vi "Init.vi"(7 "I2C #":T2=-1, 8 "error in (no error)":errorcluster, 9 "Address":T1=48 format="%02x", 10 "Session In":refnum<class "Session.lvclass">) -> (0 "error out":errorcluster, 3 "Grove I2C Matrix LED Driver Out":refnum<class "Grove I2C Matrix LED Driver.lvclass">)   [LabVIEW 2020, in "CTI-Peripheral.lvlib" / "Grove I2C Matrix LED Driver.lvclass"]
uses:
  Grove I2C Matrix LED Driver.lvclass
  CTI/I2C Connection/I2C Connection.lvclass/I2C Connection.ctl
  Grove I2C Matrix LED Driver.lvclass/Grove I2C Matrix LED Driver.ctl
  CTI/I2C Connection/I2C Connection.lvclass
  CTI/Session/Session.lvclass
  CTI/I2C Number.ctl
  CTI/CTI.lvlib
  CTI/I2C Address.ctl
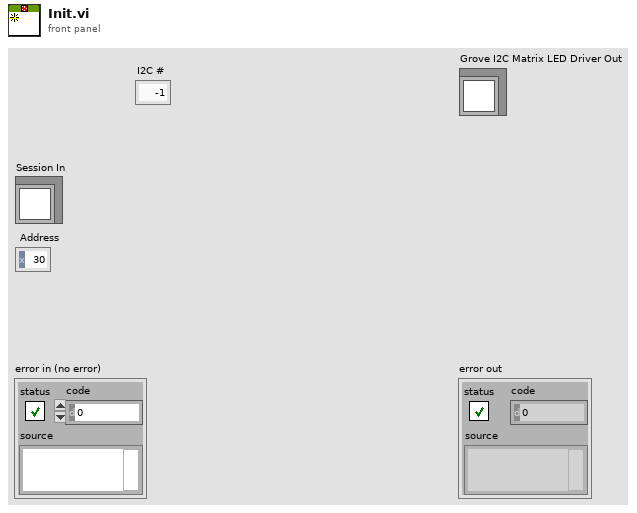
[diagram p1: front panel]
types:
  T1 = typedef "CTI.lvlib/I2C Address.ctl" = u8
  T2 = typedef "CTI.lvlib/I2C Number.ctl" = i8
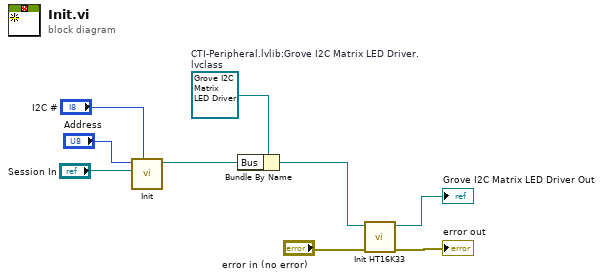
[diagram p0: block diagram]
diagram:
  w5 = refnum<class "Grove I2C Matrix LED Driver.lvclass"> refnum  # CTI-Peripheral.lvlib:Grove I2C Matrix LED Driver.lvclass
  n1 = call "Init.vi"("I2C #"="I2C #", "Session"="Session In", "Address"="Address") -> ("I2C Connection"=w9:refnum<class "I2C Connection.lvclass">)  [unwired: 7 in, 1 out]
  n2 = Bundle By Name(cluster=w5, "Bus"=w9) -> (w2:refnum<class "Grove I2C Matrix LED Driver.lvclass">)
  n3 = call "Init HT16K33.vi"("error in (no error)"="error in (no error)", "Grove I2C Matrix LED Driver.lvclass in"=w2) -> ("error out"=→"error out":errorcluster, "Grove I2C Matrix LED Driver.lvclass out"=→"Grove I2C Matrix LED Driver Out":refnum<class "Grove I2C Matrix LED Driver.lvclass">)  [unwired: 8 in]
